vi "All stations path config.vi"(10 "station idx":i32, 11 "configuration file path":path) -> (0 "error out":errorcluster, 2 "station idx":i32, 3 "configuration file path":path, 5 "paths config":T1)   [LabVIEW 2018]
uses:
  Crl defs/one state paths config.ctl
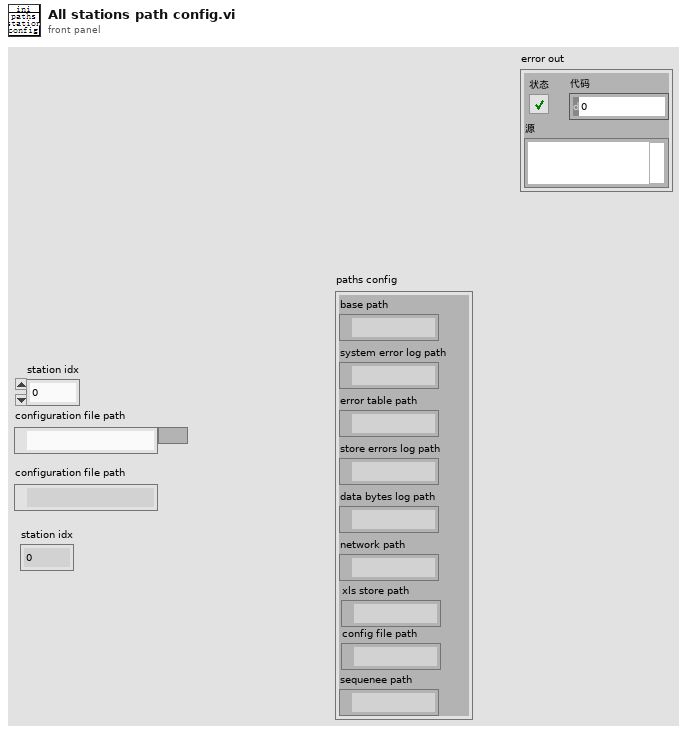
[diagram p1: front panel]
types:
  T1 = typedef "one state paths config.ctl" = cluster{"base path":path, "system error log path":path, "error table path":path, "store errors log path":path, "data bytes log path":path, "network path":path, "xls store path":path, "config file path":path, "sequenee path":path}
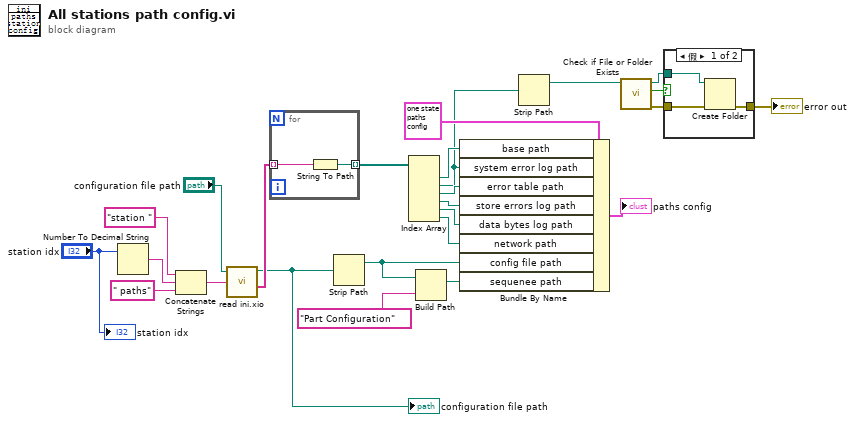
[diagram p0: block diagram]
diagram:
  n1 = Number To Decimal String(number="station idx") -> (decimal integer string=w25:string)  [unwired: 1 in]
  n2 = Concatenate Strings("station ", w25, " paths" ("string")) -> (w22:string)
  n3 = call "read ini.xio.vi"("configuration file path"="configuration file path", "Sections"=w22) -> ("configuration file path"=w4:path, "Values"=w18:string[])  [unwired: 1 in, 3 out]
  "configuration file path" <- w4
  n4 = for {
    tunnel: w18 -> [w27] mode=indexing
    tunnel: [w26] -> w11 mode=indexing
    n5 = String To Path(string=w27) -> (path=w26:path)
  }
  n6 = Strip Path(path=w4) -> (stripped path=w3:path)  [unwired: 1 out]
  n7 = Index Array(array=w11) -> (element #1=w17:path, element #2=w5:path, element #3=w16:path, element #4=w15:path, element #5=w14:path, element #6=w13:path)  [unwired: 6 in]
  n8 = Build Path(base path=w3, name or relative path="Part Configuration" ("名称或相对路径")) -> (appended path=w2:path)
  n9 = Bundle By Name(cluster=T1 {"base path"=path "", "system error log path"=path "", "error table path"=path "", "store errors log path"=path "", "data bytes log path"=path "", "network path"=path "", "xls store path"=path "", "config file path"=path "", "sequenee path"=path ""} ("paths config"), "base path"=w17, "system error log path"=w5, "error table path"=w16, "store errors log path"=w15, "data bytes log path"=w14, "network path"=w13, "config file path"=w3, "sequenee path"=w2) -> (→"paths config":T1)
  n10 = Strip Path(path=w5) -> (stripped path=w6:path)  [unwired: 1 out]
  n11 = call <vilib>:"Check if File or Folder Exists.vi"("path"=w6) -> ("error out"=w7:errorcluster, "file or folder exists?"=w9:bool, "dup path"=w8:path)  [unwired: 8 in]
  n12 = case shown="假" w9 {
    tunnel: w8 -> [w30 _]
    tunnel: [w28 w31] -> w10
    tunnel: w7 -> [w29 w31]
    frame False {
      n13 = Create Folder(path (use dialog)=w30, error in=w29) -> (error out=w28:errorcluster)  [unwired: 1 in, 2 out]
    }
    frame True {
    }
  }
  "error out" <- w10
  "station idx" <- "station idx"
